vi "wjazdczywyjazd_SubVI.vi"(5 "WE":T1(ring), 7 "czujnik brama zamkniêta":bool, 8 "czujnik laserowy \nbrama otwarta":bool, 9 "czujnik laserowy wyjazd":bool, 10 "czujnik laserowy \nwjazd":bool) -> (3 "Enum":T1(ring))   [LabVIEW 2017]
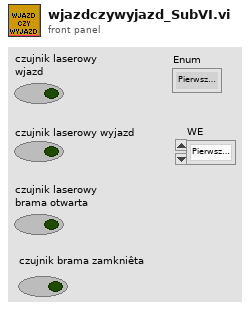
[diagram p1: front panel]
types:
  T1 = enum16{"Pierwszy wjazd", "Nikt", "Pierwszy wyjazd"}
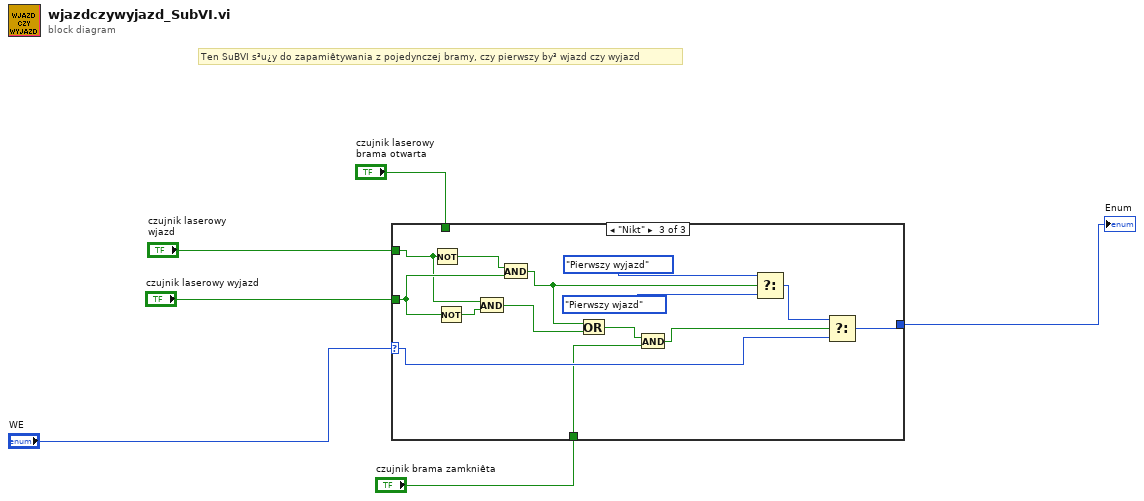
[diagram p0: block diagram]
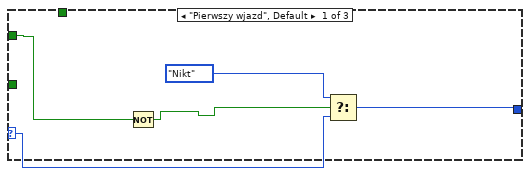
[diagram p2: hidden frame]
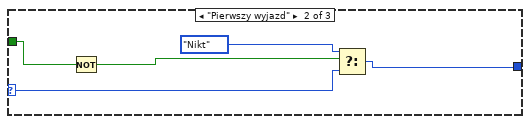
[diagram p3: hidden frame]
diagram:
  # "Ten SuBVI s³u¿y do zapamiêtywania z pojedynczej bramy, czy pierwszy by³ wjazd czy wyjazd"
  n1 = case shown="\"Nikt\"" "WE" {
    selector: "WE" -> [w9 w15 w25]
    tunnel: "czujnik laserowy \nwjazd" -> [w8 _ w20]
    tunnel: "czujnik laserowy wyjazd" -> [_ w13 w24]
    tunnel: [w11 w14 w30] -> w3
    tunnel: "czujnik laserowy \nbrama otwarta" -> [_ _ _]
    tunnel: "czujnik brama zamkniêta" -> [_ _ w18]
    frame "Pierwszy wjazd", Default {
      n2 = Not(x=w8) -> (.not. x?=w7:bool)
      n3 = Select(t=T1."Nikt", s=w7, f=w9) -> (s? t:f=w11:T1)
    }
    frame "Pierwszy wyjazd" {
      n4 = Not(x=w13) -> (.not. x?=w12:bool)
      n5 = Select(t=T1."Nikt", s=w12, f=w15) -> (s? t:f=w14:T1)
    }
    frame "Nikt" {
      n6 = Not(x=w20) -> (.not. x?=w29:bool)
      n7 = Not(x=w24) -> (.not. x?=w21:bool)
      n8 = And(x=w20, y=w21) -> (x .and. y?=w22:bool)
      n9 = And(x=w29, y=w24) -> (x .and. y?=w23:bool)
      n10 = Or(x=w23, y=w22) -> (x .or. y?=w19:bool)
      n11 = And(x=w19, y=w18) -> (x .and. y?=w17:bool)
      n12 = Select(t=T1."Pierwszy wyjazd", s=w23, f=T1."Pierwszy wjazd") -> (s? t:f=w26:T1)
      n13 = Select(t=w26, s=w17, f=w25) -> (s? t:f=w30:T1)
    }
  }
  "Enum" <- w3
